vi "Re-tag Larvae v1 (SubVI).vi"(0 "Image Size":T2={"Height"=512, "Width"=512} {"Width" step=8; "Height" step=8}, 1 "BG SUB TH":i16=20, 2 "Subtract BG":bool, 3 "BG Image":u8[][](array[numeric]), 5 "Data In":T1, 6 "Range":cluster{"Lower value":u8, "Upper value":u8}={"Lower value"=100, "Upper value"=255}, 8 "Box Side":cluster{"Low":u32, "High":u32}={"Low"=16, "High"=96}, 10 "Box W + L":cluster{"Low":u32, "High":u32}={"Low"=40, "High"=150}, 12 "Area":cluster{"Low":u32, "High":u32}={"Low"=448, "High"=1280}) -> (14 "# of Objects":i32, 16 "BBOX Array":u64[](array[numeric]), 19 "HT LOC":u64[](array[numeric]))   [LabVIEW 2015]
uses:
  Controls (HOST)/Image Size.ctl
  Controls (HOST)/Data to Disk Bundle.ctl
  <vilib>/vision/NI_Vision_Development_Module.lvlib
panel:
  out "Array":i32[](array[numeric])
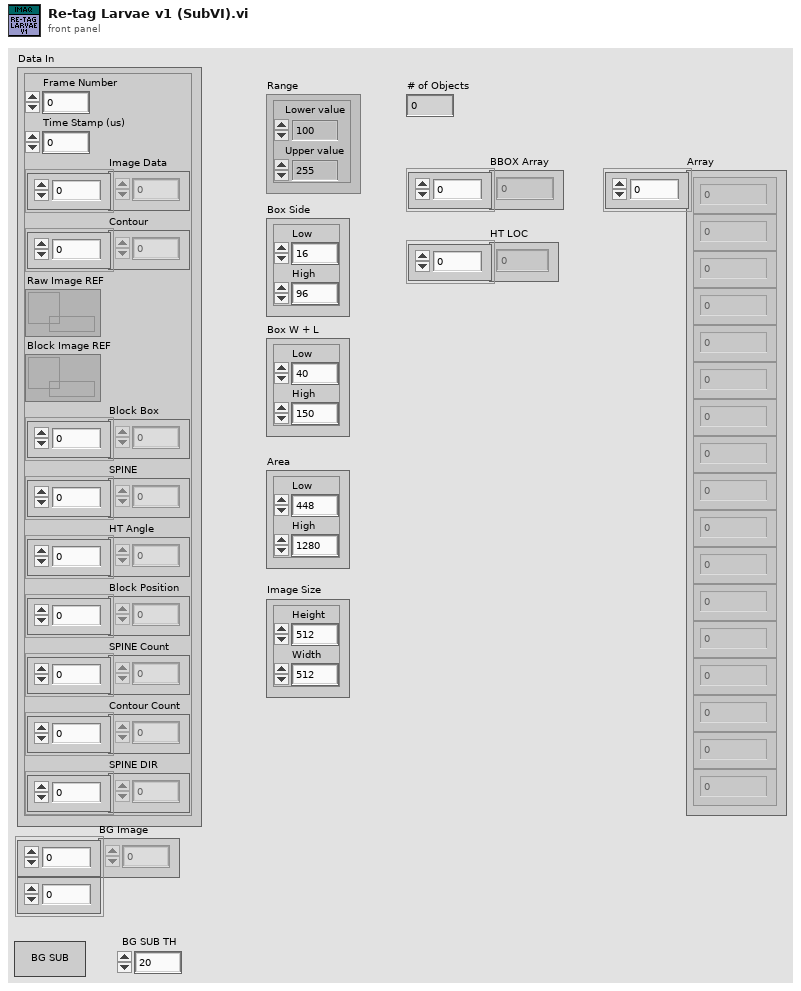
[diagram p1: front panel]
types:
  T1 = typedef "Data to Disk Bundle.ctl" = cluster{"Frame Number":u64, "Time Stamp (us)":u64, "Image Data":u64[], "Contour":u32[], "Raw Image REF":refnum<data-value>, "Block Image REF":refnum<data-value>, "Block Box":u64[], "SPINE":u32[], "HT Angle":u64[], "Block Position":u64[], "SPINE Count":u32[], "Contour Count":u32[], "SPINE DIR":u8[]}
  T2 = typedef "Image Size.ctl" = cluster{"Height":u16, "Width":u16}
  T3 = enum16{"big-endian, network order", "native, host order", "little-endian"}
  T4 = typedef "IMAQ Image.ctl" = refnum<image>
  T5 = cluster{"Area":dbl, "Number of Holes":dbl, "Bounding Rect":cluster{"Left":dbl, "Top":dbl, "Right":dbl, "Bottom":dbl}, "Center of Mass":cluster{"X":dbl, "Y":dbl}, "Orientation":dbl, "Dimensions":cluster{"Width":dbl, "Height":dbl}}[]
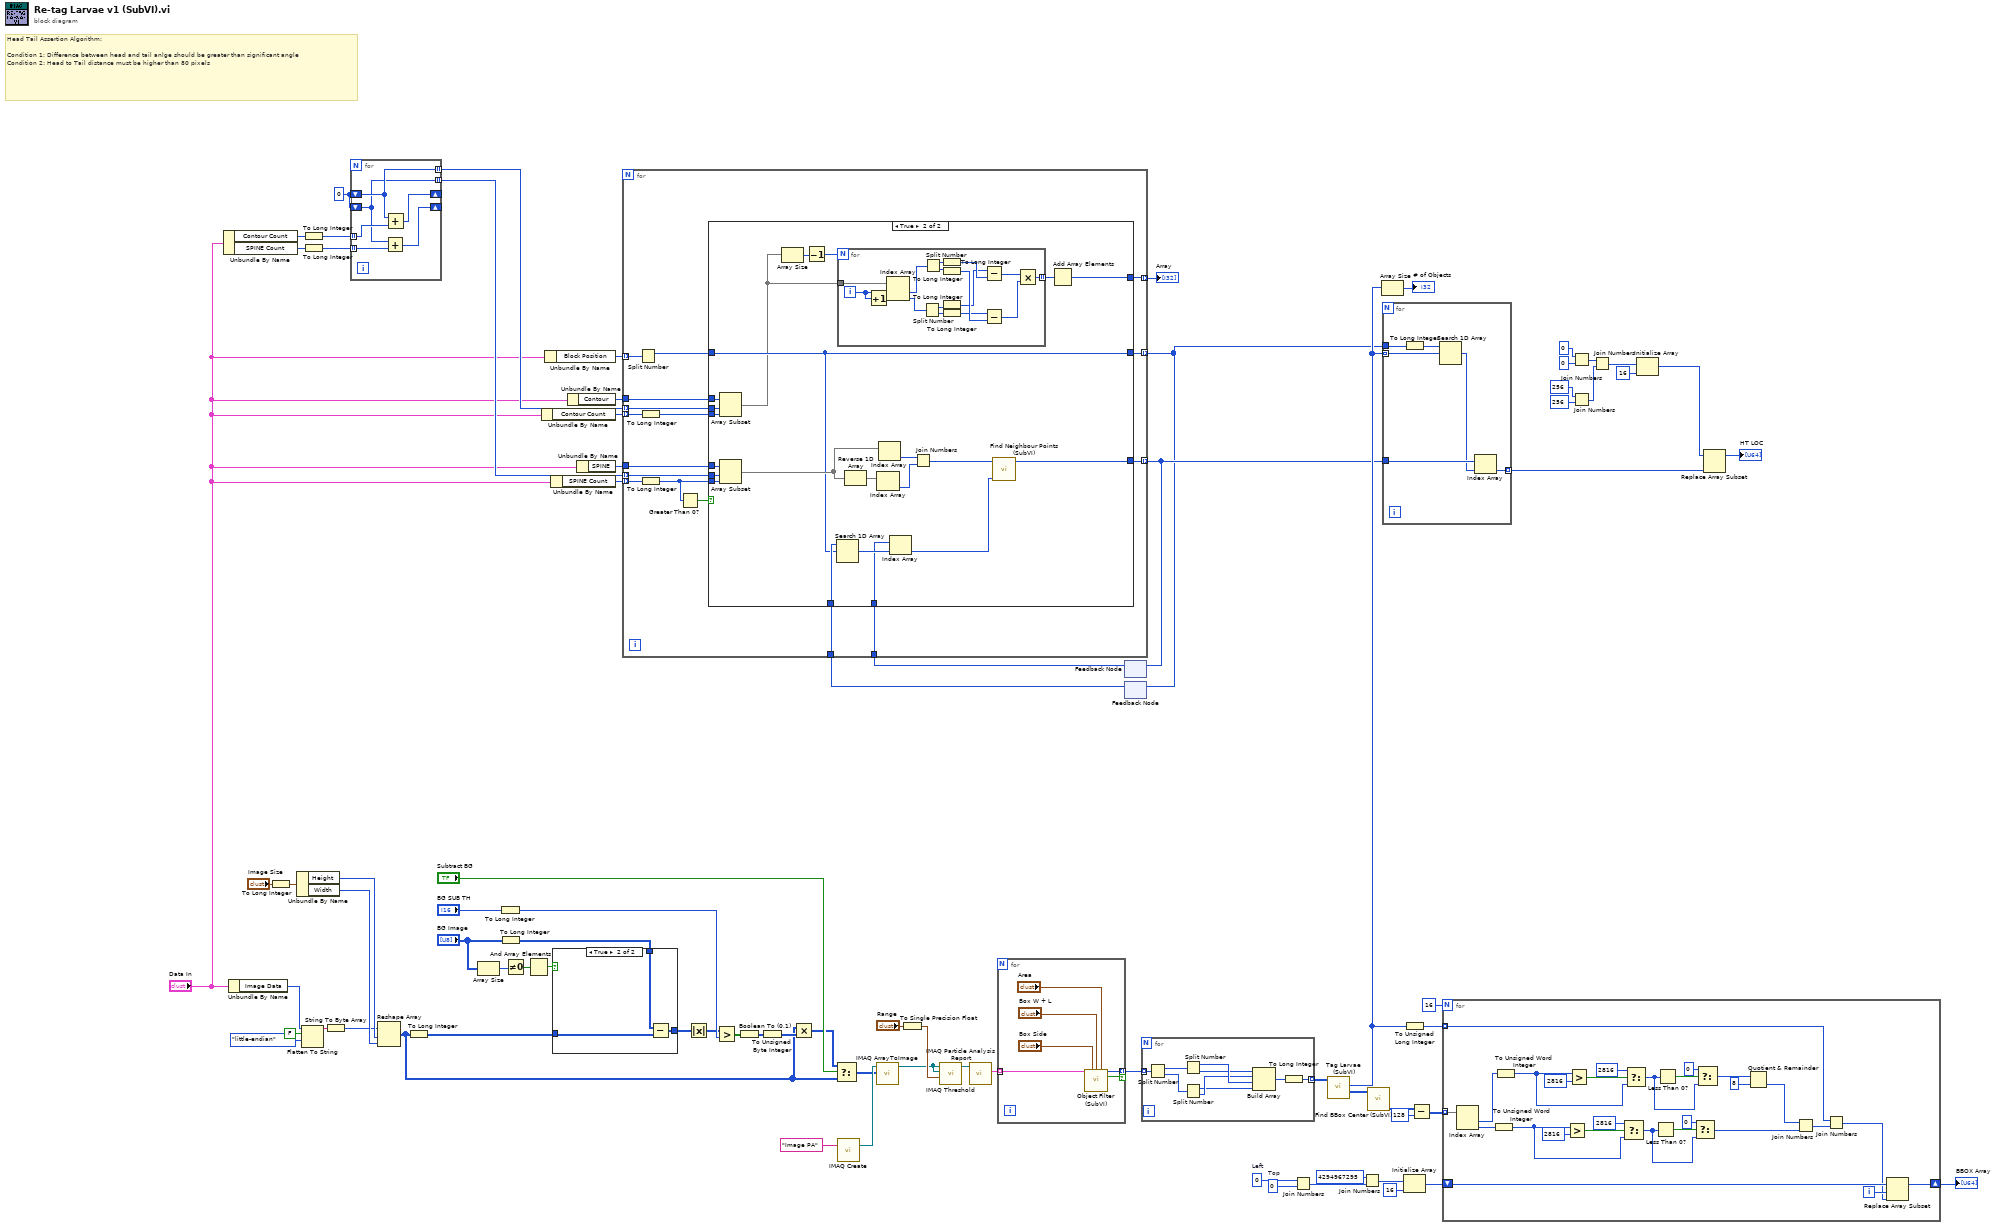
[diagram p0: block diagram]
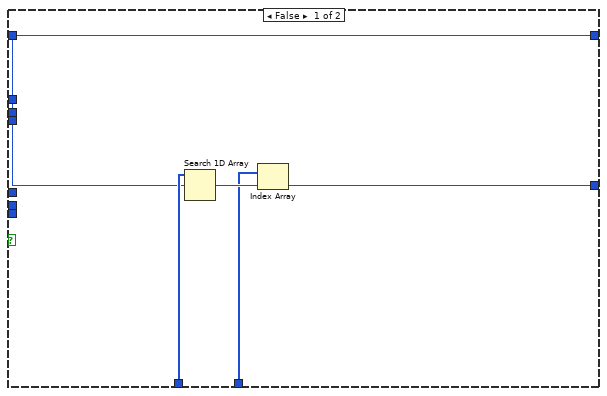
[diagram p2: hidden frame]
diagram:
  w13 = 0 ("Numeric Control")
  w63 = u16 0  # Left
  w59 = u16 0  # Top
  # "Head Tail Assertion Algorithm:\n\nCondition 1: Difference between head and tail anlge should be greater than significant angle\nCondition 2: Head to Tail distance must be higher than 80 pixels"
  n1 = Unbundle By Name("Data In") -> ("Contour Count"=w15:u32[], "SPINE Count"=w14:u32[])
  n2 = Unbundle By Name("Data In") -> ("Image Data"=w46:u64[])
  n3 = To Long Integer(number="Image Size") -> (32bit integer=w39:cluster{"Height":i32, "Width":i32})
  n4 = Unbundle By Name(w39) -> ("Height"=w41:i32, "Width"=w40:i32)
  n5 = Flatten To String(anything=w46, prepend array or string size? (T)=FALSE, byte order (0:big-endian, network order)=T3."little-endian") -> (data string=w43:string)  [unwired: 1 in, 2 out]
  n6 = To Long Integer(number=w15) -> (32bit integer=w10:i32[])
  n7 = To Long Integer(number=w14) -> (32bit integer=w11:i32[])
  n8 = String To Byte Array(string=w43) -> (unsigned byte array=w33:u8[])
  n9 = for {
    tunnel: w10 -> [w85] mode=indexing
    tunnel: w11 -> [w83] mode=indexing
    shift-right: [w86] -> _
    shift-left: w13 -> [w82]
    shift-right: [w84] -> _
    shift-left: w13 -> [w81]
    tunnel: [w82] -> w8 mode=indexing
    tunnel: [w81] -> w9 mode=indexing
    n10 = Add(x=w81, y=w83) -> (x+y=w84:i32)
    n11 = Add(x=w82, y=w85) -> (x+y=w86:i32)
  }
  n12 = Reshape Array(w33, w41, w40) -> (w16:u8[][])
  n13 = To Long Integer(number=w16) -> (32bit integer=w56:i32[][])
  n14 = Array Size(array="BG Image") -> (size(s)=w36:i32[])
  n15 = To Long Integer(number="BG SUB TH") -> (32bit integer=w47:i32)
  n16 = To Long Integer(number="BG Image") -> (32bit integer=w55:i32[][])
  n17 = Not Equal To 0?(x=w36) -> (x != 0?=w35:bool[])
  n18 = And Array Elements(Boolean array=w35) -> (logical AND=w34:bool)
  n19 = Unbundle By Name("Data In") -> ("Contour Count"=w3:u32[])
  n20 = Unbundle By Name("Data In") -> ("Block Position"=w5:u64[])
  n21 = Unbundle By Name("Data In") -> ("SPINE Count"=w4:u32[])
  n22 = case shown="True" w34 {
    tunnel: w56 -> [w87 w90]
    tunnel: w55 -> [_ w89]
    tunnel: [w87 w88] -> w54
    frame False {
    }
    frame True {
      n23 = Subtract(x=w89, y=w90) -> (x-y=w88:i32[][])
    }
  }
  n24 = Unbundle By Name("Data In") -> ("Contour"=w7:u32[])
  n25 = Unbundle By Name("Data In") -> ("SPINE"=w12:u32[])
  n26 = Absolute Value(x=w54) -> (abs(x)=w32:i32[][])
  n27 = Greater?(x=w32, y=w47) -> (0:w52:bool[][])
  n28 = Boolean To (0,1)(Boolean=w52) -> (0, 1=w51:i16[][])
  n29 = To Unsigned Byte Integer(number=w51) -> (unsigned 8bit integer=w50:u8[][])
  n30 = Multiply(x=w16, y=w50) -> (x*y=w49:u8[][])
  n31 = Select(t=w49, s="Subtract BG", f=w16) -> (s? t:f=w38:u8[][])
  n32 = call "IMAQ Create"("Image Name"="Image PA") -> ("New Image"=w72:T4)  [unwired: 4 in, 1 out]
  n33 = call "IMAQ ArrayToImage"("Image Pixels (U8)"=w38, "Image"=w72) -> ("Image Out"=w74:T4)  [unwired: 8 in, 1 out]
  n34 = To Single Precision Float(number="Range") -> (single precision float=w80:cluster{"Lower value":sgl, "Upper value":sgl})
  n35 = call "IMAQ Threshold"("Range"=w80, "Image Dst"=w74, "Image Src"=w74) -> ("Image Dst Out"=w73:T4)  [unwired: 7 in, 1 out]
  n36 = call "IMAQ Particle Analysis Report"("Image"=w73) -> ("Particle Reports (Pixels)"=w76:T5)  [unwired: 5 in, 5 out]
  n37 = for {
    tunnel: w76 -> [w92] mode=indexing
    tunnel: [w96] -> w77 mode=indexing if=w91
    n38 = call "Object Filter (SubVI).vi"("Particle Report"=w92, "Box Side"="Box Side", "Box W + L"="Box W + L", "Area"="Area") -> ("Bounding Box"=w96:u64, "Data Valid"=w91:bool)  [unwired: 10 in]
  }
  n39 = feedback #1() -> (w18:u64[])  [unwired: 1 in]
  n40 = feedback #2() -> (w20:u32[])  [unwired: 1 in]
  n41 = for {
    tunnel: w12 -> [w98]
    tunnel: [w112] -> w19 mode=indexing
    tunnel: w5 -> [w111] mode=indexing
    tunnel: w20 -> [w108]
    tunnel: w18 -> [w107]
    tunnel: w4 -> [w106] mode=indexing
    tunnel: w9 -> [w105] mode=indexing
    tunnel: w3 -> [w104] mode=indexing
    tunnel: w8 -> [w103] mode=indexing
    tunnel: w7 -> [w99]
    tunnel: [w102] -> w6 mode=indexing
    tunnel: [w97] -> w1 mode=indexing
    n42 = Split Number(x=w111) -> (hi(x)=w109:u32)  [unwired: 1 out]
    n43 = To Long Integer(number=w104) -> (32bit integer=w100:i32)
    n44 = To Long Integer(number=w106) -> (32bit integer=w101:i32)
    n45 = Greater Than 0?(x=w101) -> (x > 0?=w110:bool)
    n46 = case shown="True" w110 {
      tunnel: w98 -> [_ w139]
      tunnel: w101 -> [_ w138]
      tunnel: w105 -> [_ w137]
      tunnel: [w114 w128] -> w112
      tunnel: w109 -> [w113 w123]
      tunnel: w108 -> [w117 w134]
      tunnel: w107 -> [w115 w133]
      tunnel: w100 -> [_ w126]
      tunnel: w103 -> [_ w125]
      tunnel: w99 -> [_ w124]
      tunnel: [w113 w123] -> w102
      tunnel: [_ w118] -> w97
      frame False {
        n47 = Search 1D Array(1D array=w117, element=w113) -> (index of element=w116:i32)  [unwired: 1 in]
        n48 = Index Array(array=w115, index=w116) -> (element=w114:u64)
      }
      frame True {
        n49 = Array Subset(array=w124, index=w125, length=w126) -> (w120:u32[])
        n50 = Array Subset(array=w139, index=w137, length=w138) -> (w127:u32[])
        n51 = Array Size(array=w120) -> (size(s)=w122:i32)
        n52 = Decrement(x=w122) -> (x-1=w121:i32)
        n53 = Search 1D Array(1D array=w134, element=w123) -> (index of element=w135:i32)  [unwired: 1 in]
        n54 = for {
          N: w121 -> [_]
          tunnel: w120 -> [w155]
          tunnel: [w148] -> w119 mode=indexing
          i -> [w141]
          n55 = Increment(x=w141) -> (x+1=w140:i32)
          n56 = Index Array(array=w155, index #1=w141, index #2=w140) -> (element #1=w147:u32, element #2=w146:u32)
          n57 = Split Number(x=w146) -> (hi(x)=w153:u16, lo(x)=w151:u16)
          n58 = Split Number(x=w147) -> (hi(x)=w154:u16, lo(x)=w152:u16)
          n59 = To Long Integer(number=w154) -> (32bit integer=w145:i32)
          n60 = To Long Integer(number=w152) -> (32bit integer=w144:i32)
          n61 = To Long Integer(number=w153) -> (32bit integer=w143:i32)
          n62 = To Long Integer(number=w151) -> (32bit integer=w142:i32)
          n63 = Subtract(x=w143, y=w145) -> (x-y=w150:i32)
          n64 = Subtract(x=w142, y=w144) -> (x-y=w149:i32)
          n65 = Multiply(x=w150, y=w149) -> (x*y=w148:i32)
        }
        n66 = Reverse 1D Array(array=w127) -> (reversed array=w136:u32[])
        n67 = Index Array(array=w136) -> (element=w131:u32)  [unwired: 1 in]
        n68 = Index Array(array=w127) -> (element=w130:u32)  [unwired: 1 in]
        n69 = Index Array(array=w133, index=w135) -> (element=w129:u64)
        n70 = Join Numbers(hi=w130, lo=w131) -> ((hi.lo)=w132:u64)
        n71 = call "Find Neighbour Points (SubVI).vi"("Previous HT Position"=w129, "Current HT Position"=w132) -> ("Neighbor Point"=w128:u64)  [unwired: 9 in]
        n72 = Add Array Elements(numeric array=w119) -> (sum=w118:i32)
      }
    }
  }
  "Array" <- w1
  n73 = feedback-in #1(w19) -> ()
  n74 = feedback-in #2(w6) -> ()
  n75 = for {
    tunnel: w77 -> [w164] mode=indexing
    tunnel: [w156] -> w57 mode=indexing
    n76 = Split Number(x=w164) -> (hi(x)=w163:u32, lo(x)=w162:u32)
    n77 = Split Number(x=w163) -> (hi(x)=w161:u16, lo(x)=w160:u16)
    n78 = Split Number(x=w162) -> (hi(x)=w158:u16, lo(x)=w159:u16)
    n79 = Build Array(w160, w159, w161, w158) -> (w157:u16[])
    n80 = To Long Integer(number=w157) -> (32bit integer=w156:i32[])
  }
  n81 = Join Numbers(hi=w63, lo=w59) -> ((hi.lo)=w60:u32)
  n82 = call "Tag Larvae (SubVI).vi"("Array in"=w57) -> ("Bounding Box"=w66:i32[][], "Current ID"=w31:i32[])  [unwired: 8 in, 1 out]
  n83 = Join Numbers(hi=u32 4294967295, lo=w60) -> ((hi.lo)=w61:u64)
  n84 = call "Find BBox Center (SubVI).vi"("BBox Array In"=w66) -> ("Center Array"=w67:i32[][])  [unwired: 9 in, 1 out]
  n85 = Array Size(array=w31) -> (size(s)=→"# of Objects":i32)
  n86 = for {
    tunnel: w31 -> [w169] mode=indexing
    tunnel: w6 -> [w170]
    tunnel: w19 -> [w167]
    tunnel: [w166] -> w22 mode=indexing
    n87 = To Long Integer(number=w170) -> (32bit integer=w168:i32[])
    n88 = Search 1D Array(1D array=w168, element=w169) -> (index of element=w165:i32)  [unwired: 1 in]
    n89 = Index Array(array=w167, index=w165) -> (element=w166:u64)
  }
  n90 = To Unsigned Long Integer(number=w31) -> (unsigned 32bit integer=w79:u32[])
  n91 = Initialize Array(w61, 16 ("dimension size")) -> (w64:u64[])
  n92 = Subtract(x=w67, y=128) -> (x-y=w68:i32[][])
  n93 = for {
    N: 16 -> [_]
    shift-right: [w196] -> w70
    shift-left: w64 -> [w197]
    tunnel: w68 -> [w194] mode=indexing
    tunnel: w79 -> [w172] mode=indexing
    i -> [w195]
    n94 = Index Array(array=w194) -> (element #1=w176:i32, element #2=w177:i32)  [unwired: 2 in]
    n95 = To Unsigned Word Integer(number=w177) -> (unsigned 16bit integer=w187:u16)
    n96 = To Unsigned Word Integer(number=w176) -> (unsigned 16bit integer=w186:u16)
    n97 = Greater?(x=w187, y=u16 2816) -> (0:w193:bool)
    n98 = Greater?(x=w186, y=u16 2816) -> (0:w180:bool)
    n99 = Select(t=u16 2816 ("y"), s=w193, f=w187) -> (s? t:f=w189:u16)
    n100 = Select(t=u16 2816 ("y"), s=w180, f=w186) -> (s? t:f=w184:u16)
    n101 = Less Than 0?(x=w189) -> (x < 0?=w190:bool)
    n102 = Less Than 0?(x=w184) -> (x < 0?=w183:bool)
    n103 = Select(t=u16 0 ("y"), s=w190, f=w189) -> (s? t:f=w174:u16)
    n104 = Select(t=u16 0 ("y"), s=w183, f=w184) -> (s? t:f=w179:u16)
    n105 = Quotient & Remainder(x=w179, y=u16 8) -> (floor(x/y)=w175:u16)  [unwired: 1 out]
    n106 = Join Numbers(hi=w175, lo=w174) -> ((hi.lo)=w173:u32)
    n107 = Join Numbers(hi=w172, lo=w173) -> ((hi.lo)=w171:u64)
    n108 = Replace Array Subset(array=w197, new element=w171, index=w195) -> (w196:u64[])
  }
  "BBOX Array" <- w70
  n109 = Join Numbers(hi=u16 0 ("Numeric Control"), lo=u16 0 ("Numeric Control")) -> ((hi.lo)=w26:u32)
  n110 = Join Numbers(hi=u16 256 ("Numeric Control"), lo=u16 256 ("Numeric Control")) -> ((hi.lo)=w25:u32)
  n111 = Join Numbers(hi=w26, lo=w25) -> ((hi.lo)=w24:u64)
  n112 = Initialize Array(w24, 16 ("dimension size")) -> (w17:u64[])
  n113 = Replace Array Subset(array=w17, new element=w22) -> (→"HT LOC":u64[])  [unwired: 1 in]
